vi "PV ActiveLine - SwitchingFunctionStatus.vi"(8 "Fehler (Eingang)":errorcluster, 11 "Referenz in":refnum<visa-resource-name>) -> (0 "Cluster (Ausgang)":errorcluster, 1 "Set Point 3":u8(ring)=3 items=["off", "on"], 2 "Set Point 2":u8(ring)=3 items=["off", "on"], 3 "Referenz out":refnum<visa-resource-name>, 4 "Set Point 4":u8(ring)=3 items=["off", "on"], 5 "Set Point 1":u8(ring)=3 items=["off", "on"])   [LabVIEW 2013, in "PV ActiveLine.lvlib"]
doc: "SPS - Switching Function Status\n\nReceive: a,b,c,d\n\nStatus switching function 1,\na =\n0 –> Off\n1 –> On\nStatus switching function 2,\nb =\n0 –> Off\n1 –> On\nStatus switching function 3,\nc =\n0 –> Off\n1 –> On\nStatus switching function 4,\nd =\n0 –> Off\n1 –> On"
uses:
  <instrlib>/PV ActiveLine/PV ActiveLine.lvlib
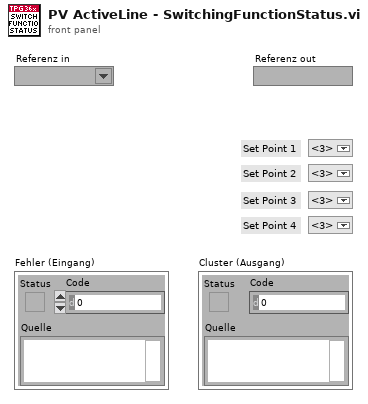
[diagram p1: front panel]
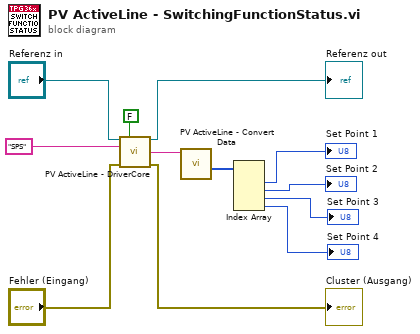
[diagram p0: block diagram]
diagram:
  n1 = call <instrlib>:"PV ActiveLine - DriverCore.vi"("Referenz in"="Referenz in", "Write/Read"=FALSE, "Command"="SPS", "Fehler (Eingang)"="Fehler (Eingang)") -> ("Referenz out"=→"Referenz out":refnum<visa-resource-name>, "String Out"=w6:string, "Cluster (Ausgang)"=→"Cluster (Ausgang)":errorcluster)  [unwired: 9 in]
  n2 = call <instrlib>:"PV ActiveLine - Convert Data.vi"("String in"=w6) -> ("Integer Out"=w5:i32[])  [unwired: 7 in, 3 out]
  n3 = Index Array(array=w5) -> (element #1=→"Set Point 1":i32, element #2=→"Set Point 2":i32, element #3=→"Set Point 3":i32, element #4=→"Set Point 4":i32)  [unwired: 4 in]
